vi "TODO.vi"(8 "error in (no error)":errorcluster, 11 "Message":string) -> (0 "error out":errorcluster)   [LabVIEW 2011]
uses:
  030 - EVENTS/03 - ToMessageHandlerProcess/enumMessageCriticity.ctl
  090 - ERRORS/Ctrls/enumLogAndView.ctl
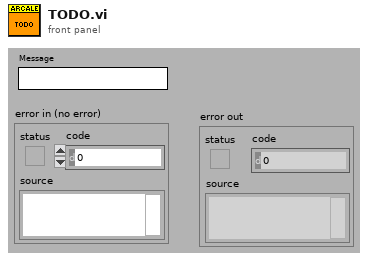
[diagram p1: front panel]
types:
  T1 = typedef "enumLogAndView.ctl" = enum16{"Log only", "Log and view"}
  T2 = typedef "enumMessageCriticity.ctl" = enum16{"No error", "Info", "Warning", "Error", "Fatal error"}
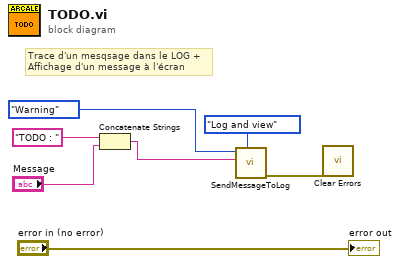
[diagram p0: block diagram]
diagram:
  # "Trace d'un mesqsage dans le LOG +\nAffichage d'un message à l'écran"
  n1 = Concatenate Strings("TODO : ", "Message") -> (w4:string)
  n2 = call "SendMessageToLog.vi"("Log and view ?"=enumLogAndView."Log and view", "Message"=w4, "Criticity"=enumMessageCriticity."Warning") -> ("error out"=w2:errorcluster)  [unwired: 8 in]
  n3 = call <vilib>:"Clear Errors.vi"("error in (no error)"=w2) -> ()  [unwired: 6 in, 1 out]
  "error out" <- "error in (no error)"
